vi "DB to Vapor Pressure.vi"(1 "Dry Bulb Temp [DegF]":dbl) -> (0 "Vapor Pressure [kPa]":dbl)   [LabVIEW 2020]
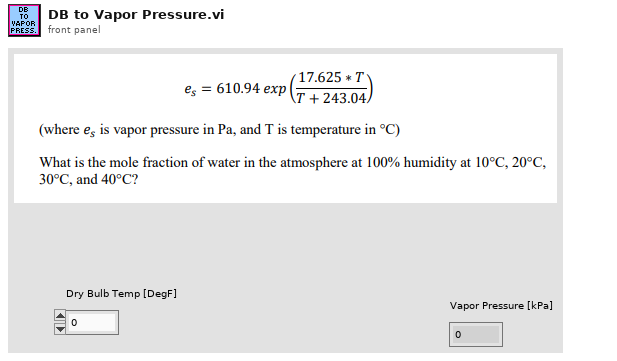
[diagram p1: front panel]
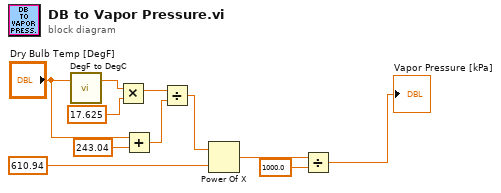
[diagram p0: block diagram]
diagram:
  n1 = call "DegF to DegC.vi"("Input Temperature in Fahrenheit"="Dry Bulb Temp [DegF]") -> ("Output Temperature in Celcius"=w10:dbl)  [unwired: 1 in, 1 out]
  n2 = Multiply(x=w10, y=17.625) -> (x*y=w8:dbl)
  n3 = Add(x="Dry Bulb Temp [DegF]", y=243.04) -> (x+y=w7:dbl)
  n4 = Divide(x=w8, y=w7) -> (x/y=w4:dbl)
  n5 = Power Of X(1:610.94 ("y"), 2:w4) -> (0:w3:dbl)
  n6 = Divide(x=w3, y=1000.0) -> (x/y=→"Vapor Pressure [kPa]":dbl)
